vi "QrCodeBuild-Gma.vi"(2 "有边缘?(T)":bool=TRUE, 3 "ErrorCorrectLevel":i32(ring) items=["L", "M", "Q", "H"], 4 "Scale(4)":u8=4, 5 "Text":string="31S5106            W84B9L004        20180419SBDCNMR-JE-70B                      0001") -> (1 "out Array":bool[][](array[boolean]))   [LabVIEW 2018]
uses:
  Gma.QrCodeNet.Encoding.dll
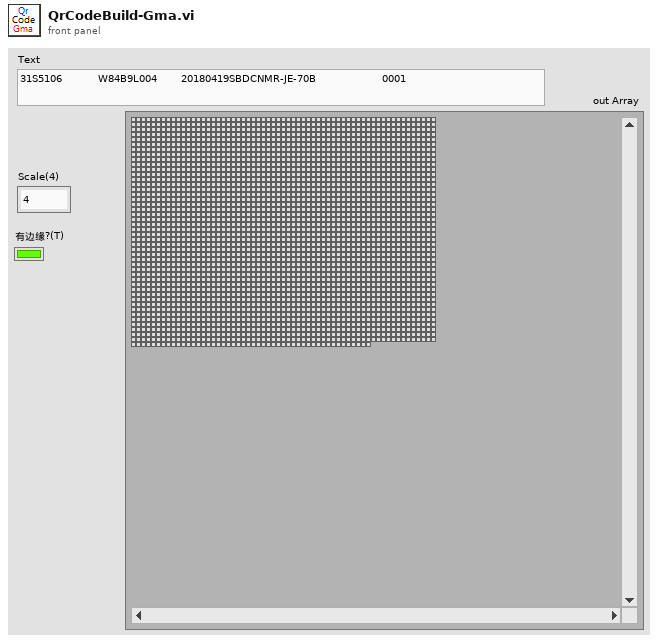
[diagram p1: front panel]
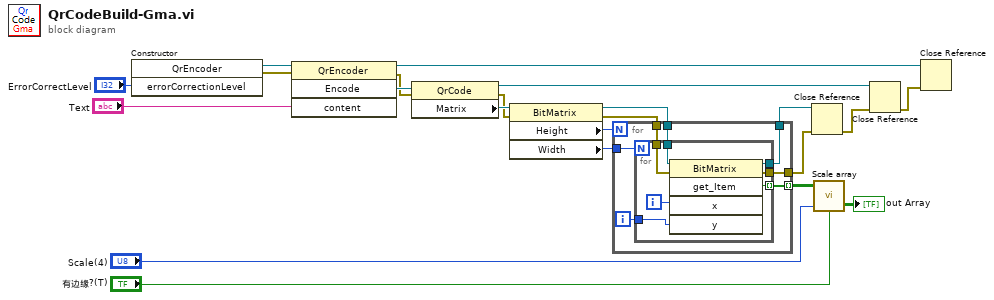
[diagram p0: block diagram]
diagram:
  n1 = constructor class="QrEncoder"("errorCorrectionLevel"="ErrorCorrectLevel") -> (reference out=w15:refnum<k24>, error out=w16:errorcluster)  [unwired: 3 in, 2 out]
  n2 = invoke class="QrEncoder" method="Encode"(reference=w15, error in=w16, "content"="Text") -> (reference out=w13:refnum<k24>, error out=w9:errorcluster, "Encode"=w14:refnum<k24>)  [unwired: 1 in, 1 out]
  n3 = property class="QrCode"(reference=w14, error in=w9) -> (reference out=w19:refnum<k24>, error out=w8:errorcluster, "Matrix"=w10:refnum<k24>)
  n4 = property class="BitMatrix"(reference=w10, error in=w8) -> (reference out=w6:refnum<k24>, error out=w5:errorcluster, "Height"=w12:i32, "Width"=w11:i32)
  n5 = for {
    N: w12 -> [_]
    tunnel: w11 -> [w29]
    tunnel: [w27] -> w7 mode=indexing
    tunnel: [w26] -> w4
    tunnel: w6 -> [w25]
    tunnel: [w24] -> w3
    tunnel: w5 -> [w23]
    i -> [w28]
    n6 = for {
      N: w29 -> [_]
      tunnel: w28 -> [w35]
      tunnel: [w34] -> w27 mode=indexing
      tunnel: [w33] -> w26
      tunnel: w25 -> [w32]
      tunnel: [w31] -> w24
      tunnel: w23 -> [w30]
      i -> [w36]
      n7 = invoke class="BitMatrix" method="get_Item"(reference=w32, error in=w30, "x"=w36, "y"=w35) -> (reference out=w33:refnum<k24>, error out=w31:errorcluster, "get_Item"=w34:bool)  [unwired: 1 in, 2 out]
    }
  }
  n8 = Close Reference(reference=w4, error in (no error)=w3) -> (error out=w18:errorcluster)
  n9 = call "Scale array.vi"("有边缘？"="有边缘?(T)", "Scale"="Scale(4)", "in Array"=w7) -> ("out Array"=→"out Array":bool[][])  [unwired: 1 in, 1 out]
  n10 = Close Reference(reference=w19, error in (no error)=w18) -> (error out=w17:errorcluster)
  n11 = Close Reference(reference=w13, error in (no error)=w17) -> ()  [unwired: 1 out]
